vi "GetMatlabTemp.vi"(6 "IgnoreContainerName":bool=TRUE, 8 "error in (no error)":errorcluster, 9 "Value Tp Update (or type)":variant, 10 "index in":dbl, 11 "ExpID":string) -> (0 "error out":errorcluster, 2 "Matlab param data":T1[](array[typedef]), 3 "Value":variant)   [LabVIEW 2017]
uses:
  Types/MatlabDataBundle.ctl
  Types/MatlabDataType.ctl
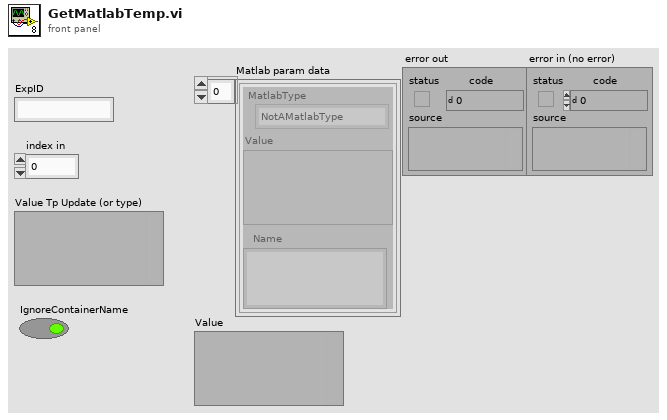
[diagram p1: front panel]
types:
  T1 = typedef "MatlabDataBundle.ctl" = cluster{"MatlabType":T2, "Value":variant, "Name":string}
  T2 = typedef "MatlabDataType.ctl" = enum16{"NotAMatlabType", "Real", "Complex", "String", "Boolean"}
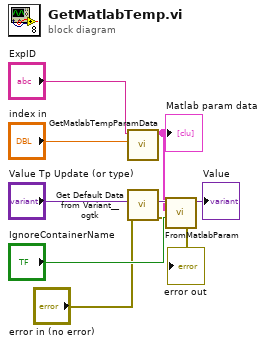
[diagram p0: block diagram]
diagram:
  n1 = call "GetMatlabTempParamData.vi"("index"="index in", "ExperimentID"="ExpID") -> ("Matlab param data"=w5:T1[])  [unwired: 9 in]
  "Matlab param data" <- w5
  n2 = call <userlib>:"Get Default Data from Variant__ogtk.vi"("error in (no error)"="error in (no error)", "Variant"="Value Tp Update (or type)") -> ("error out"=→"error out":errorcluster, "Default VData"=w7:variant)  [unwired: 8 in]
  n3 = call "FromMatlabParam.vi"("IgnoreContainerName"="IgnoreContainerName", "Matlab Param Data"=w5, "Type (or value to update)"=w7) -> ("Value"=→"Value":variant)  [unwired: 8 in]
